vi "Plot SJ Datafile.vi"(11 "File Path Control":path) -> ()   [LabVIEW 2011]
uses:
  <vilib>/Utility/file.llb/Read From Spreadsheet File (string).vi
  <vilib>/Utility/file.llb/Read From Spreadsheet File (DBL).vi
  <vilib>/Analysis/NI_AALBase.lvlib
panel:
  out "Fmax":dbl[](array[numeric])
  in  "Sort?":bool
  out "Selected Data SD":dbl format="%.2e"
  out "All Data SD":dbl format="%.2e"
  out "All Data":cluster{dbl[], dbl[]}[](graph)
  in  "Disc ID List":i32[](listbox)
  out "Selected Data":cluster{dbl[], dbl[]}[](graph)
  # "C:\\EnFlo_Data_Local\\2012\\Aero_Tunnel\\Nick_Martin\\Results_Post_Processed\\SJ_In_RP_Test_I_xls_Mean_Data\\Phase Pressure _deg_.xls"
  # "C:\\EnFlo_Data_Local\\2012\\Aero_Tunnel\\Nick_Martin\\Results_Post_Processed\\SJ_In_RP_Test_I_xls_Mean_Data\\RMS Current _A_.xls"
  # "C:\\EnFlo_Data_Local\\2012\\Aero_Tunnel\\Nick_Martin\\Results_Post_Processed\\SJ_In_RP_Test_I_xls_Mean_Data\\RMS Pressure _Pa_.xls"
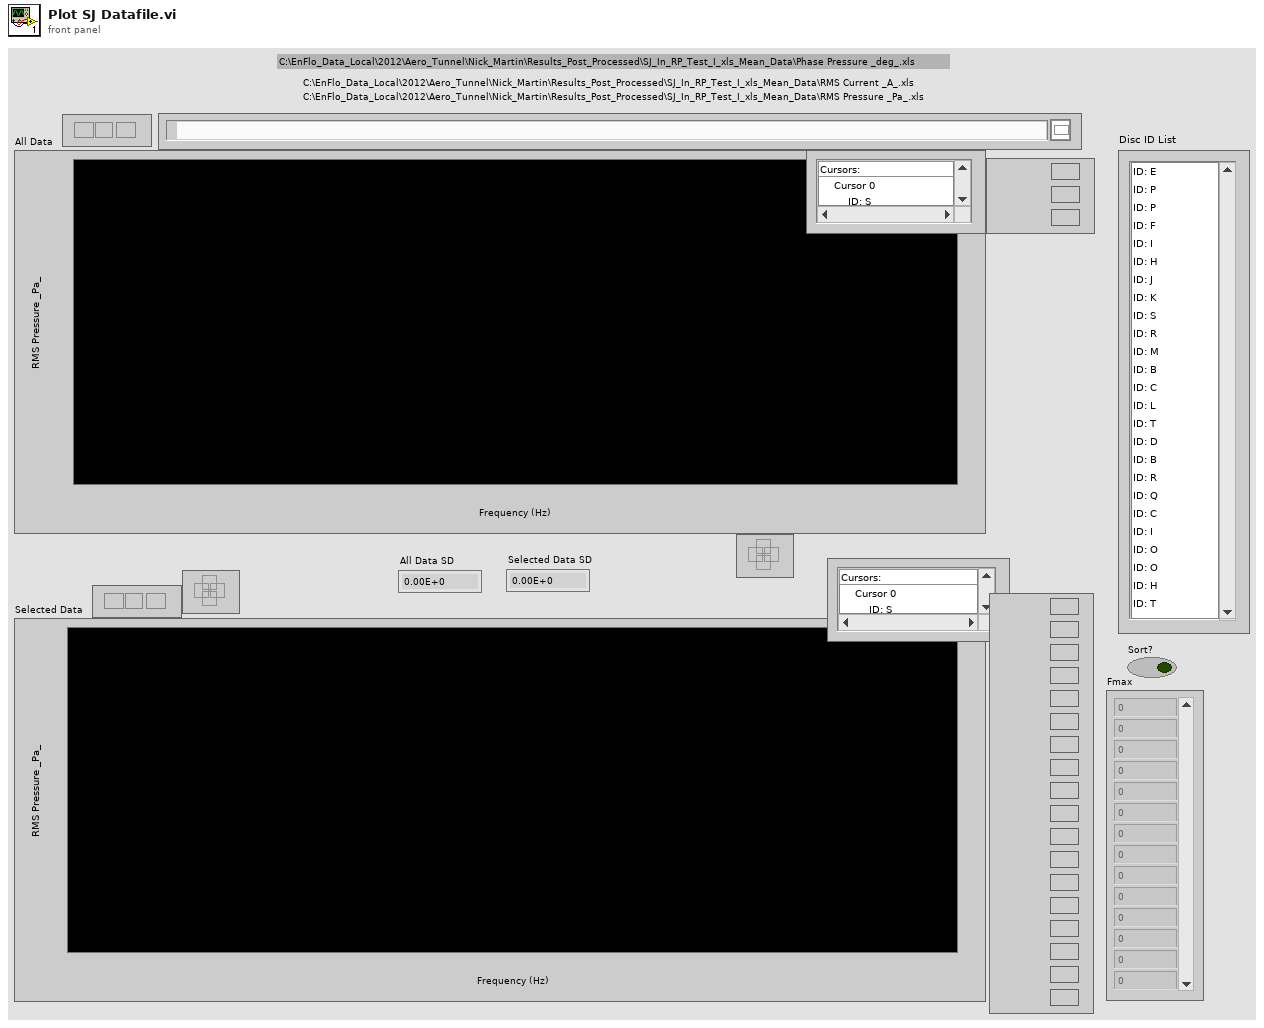
[diagram p1: front panel]
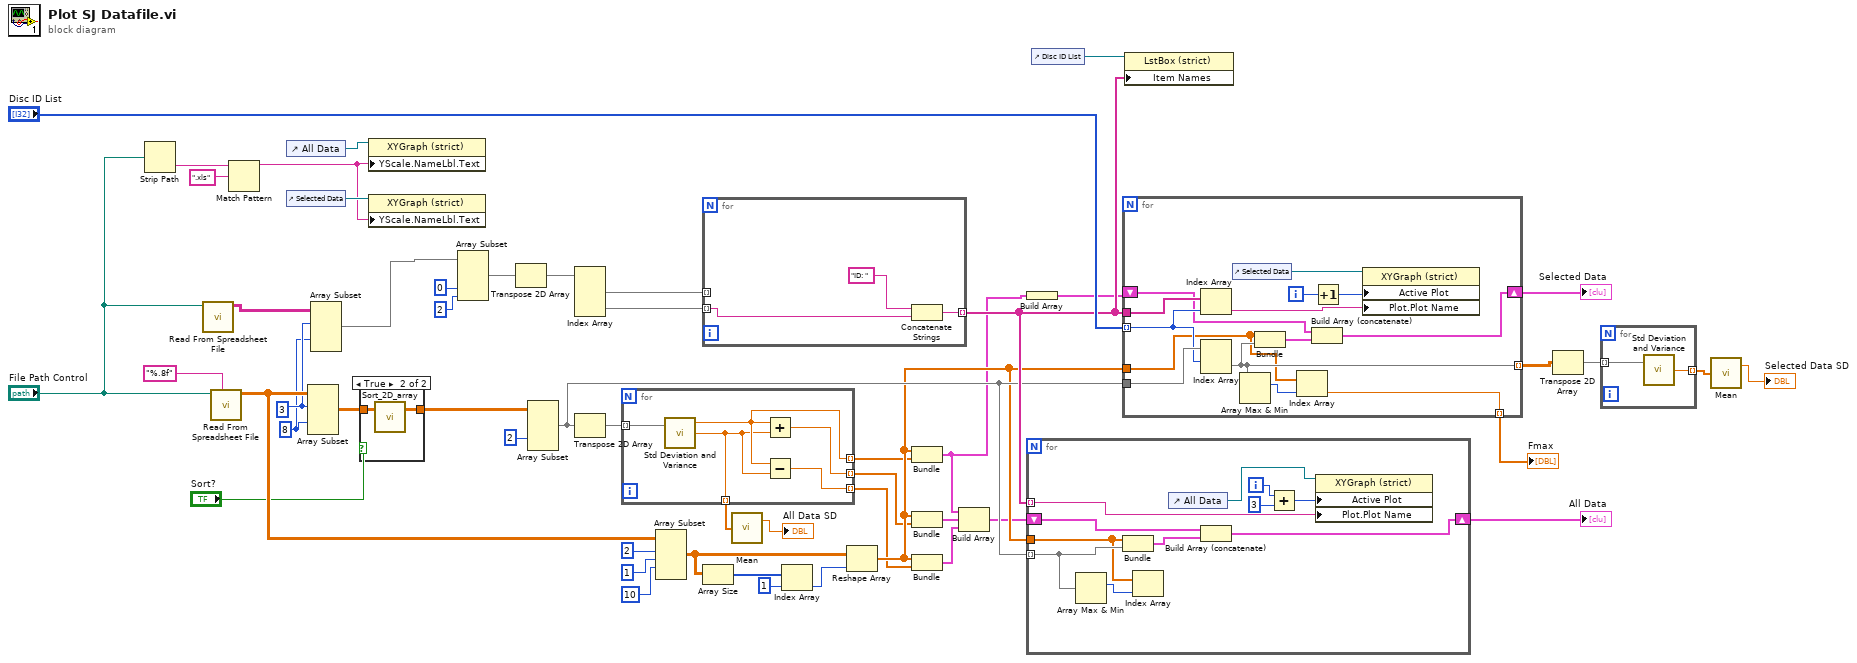
[diagram p0: block diagram]
diagram:
  w8 = 8 ("index")
  w9 = 3 ("index")
  n1 = Strip Path(path="File Path Control") -> (name=w32:string)  [unwired: 1 out]
  n2 = call-poly <vilib>:"Read From Spreadsheet File.vi"("file path (dialog if empty)"="File Path Control") -> ("all rows"=w7:string[][])  [unwired: 6 in, 4 out]
  n3 = call-poly <vilib>:"Read From Spreadsheet File.vi"("format (%.3f)"="%.8f", "file path (dialog if empty)"="File Path Control") -> ("all rows"=w44:dbl[][])  [unwired: 5 in, 4 out]
  n4 = Match Pattern(string=w32, regular expression=".xls") -> (before substring=w28:string)  [unwired: 1 in, 3 out]
  n5 = control-ref of="All Data"() -> (w30:refnum<vi>)
  n6 = control-ref of="Selected Data"() -> (w29:refnum<vi>)
  n7 = Array Subset(array=w44, index (row)=w9, index (col)=w8) -> (w42:dbl[][])  [unwired: 2 in]
  n8 = Array Subset(array=w7, index (row)=w9, index (col)=w8) -> (w5:string[][])  [unwired: 2 in]
  n9 = case shown="True" "Sort?" {
    tunnel: w42 -> [w53 w55]
    tunnel: [w53 w54] -> w4
    frame False {
    }
    frame True {
      n10 = call "Sort_2D_array.vi"("unsorted array"=w55) -> ("sorted array"=w54:dbl[][])  [unwired: 1 in, 1 out]
    }
  }
  n11 = property class="XYGraph (strict)"(reference=w30, "YScale.NameLbl.Text"=w28) -> ()  [unwired: 1 in, 2 out]
  n12 = property class="XYGraph (strict)"(reference=w29, "YScale.NameLbl.Text"=w28) -> ()  [unwired: 1 in, 2 out]
  n13 = Array Subset(array=w5, index (col)=0 ("index"), length (col)=2 ("length")) -> (w39:string[][])  [unwired: 2 in]
  n14 = Transpose 2D Array(2D array=w39) -> (transposed array=w43:string[][])
  n15 = Array Subset(array=w4, index (col)=2 ("index")) -> (w27:dbl[][])  [unwired: 3 in]
  n16 = Index Array(array=w43) -> (element #1=w3:string[], element #2=w2:string[])  [unwired: 4 in]
  n17 = Transpose 2D Array(2D array=w27) -> (transposed array=w26:dbl[][])
  n18 = for {
    tunnel: w26 -> [w60] mode=indexing
    tunnel: [w58] -> w24 mode=indexing
    tunnel: [w59] -> w23 mode=indexing
    tunnel: [w57] -> w22 mode=indexing
    tunnel: [w56] -> w18 mode=indexing
    n19 = call <vilib>:"Std Deviation and Variance.vi"("X"=w60) -> ("mean"=w58:dbl, "standard deviation"=w56:dbl)  [unwired: 1 in, 1 out]
    n20 = Add(x=w58, y=w56) -> (x+y=w59:dbl)
    n21 = Subtract(x=w58, y=w56) -> (x-y=w57:dbl)
  }
  n22 = Array Subset(array=w44, index (row)=2 ("index"), length (row)=1 ("length"), index (col)=10 ("index")) -> (w48:dbl[][])  [unwired: 1 in]
  n23 = for {
    tunnel: w2 -> [w61] mode=indexing
    tunnel: [w62] -> w34 mode=indexing
    tunnel: w3 -> [_] mode=indexing
    n24 = Concatenate Strings("ID: " ("string"), w61) -> (w62:string)
  }
  n25 = Array Size(array=w48) -> (size(s)=w47:i32[])
  n26 = call <vilib>:"Mean.vi"("X"=w18) -> ("mean"=→"All Data SD":dbl)  [unwired: 1 out]
  n27 = Index Array(array=w47, index=1) -> (element=w45:i32)
  n28 = Reshape Array(w48, w45) -> (w25:dbl[])
  n29 = Bundle(w25, w24) -> (w12:cluster{dbl[], dbl[]})  [unwired: 1 in]
  n30 = Bundle(w25, w23) -> (w21:cluster{dbl[], dbl[]})  [unwired: 1 in]
  n31 = Bundle(w25, w22) -> (w20:cluster{dbl[], dbl[]})  [unwired: 1 in]
  n32 = Build Array(w12, w21, w20) -> (w19:cluster{dbl[], dbl[]}[])
  n33 = Build Array(w12) -> (w11:cluster{dbl[], dbl[]}[])
  n34 = for {
    tunnel: w25 -> [w65]
    tunnel: w27 -> [w66] mode=indexing
    shift-right: [w72] -> w33
    shift-left: w19 -> [w71]
    tunnel: w34 -> [w70] mode=indexing
    i -> [w73]
    n35 = Array Max & Min(array=w66) -> (max index (indices)=w64:i32)  [unwired: 3 out]
    n36 = Bundle(w65, w66) -> (w74:cluster{dbl[], dbl[]})  [unwired: 1 in]
    n37 = Index Array(array=w65, index=w64) -> ()  [unwired: 1 out]
    n38 = control-ref of="All Data"() -> (w69:refnum<vi>)
    n39 = Build Array (concatenate)(w71, w74) -> (w72:cluster{dbl[], dbl[]}[])
    n40 = Add(x=w73, y=3) -> (x+y=w68:i32)
    n41 = property class="XYGraph (strict)"(reference=w69, "Active Plot"=w68, "Plot.Plot Name"=w70) -> ()  [unwired: 1 in, 2 out]
  }
  "All Data" <- w33
  n42 = control-ref of="Disc ID List"() -> (w37:refnum<vi>)
  n43 = for {
    tunnel: "Disc ID List" -> [w84] mode=indexing
    tunnel: w25 -> [w76]
    tunnel: w27 -> [w88]
    tunnel: w34 -> [w85]
    shift-right: [w82] -> w35
    shift-left: w11 -> [w81]
    tunnel: [w77] -> w15 mode=indexing
    tunnel: [w75] -> w1 mode=indexing
    i -> [w80]
    n44 = Index Array(array=w85, index=w84) -> (element=w83:string)
    n45 = Index Array(array=w88, index (row)=w84) -> (element=w77:dbl[])  [unwired: 1 in]
    n46 = control-ref of="Selected Data"() -> (w86:refnum<vi>)
    n47 = Array Max & Min(array=w77) -> (max index (indices)=w78:i32)  [unwired: 3 out]
    n48 = Bundle(w76, w77) -> (w87:cluster{dbl[], dbl[]})  [unwired: 1 in]
    n49 = Index Array(array=w76, index=w78) -> (element=w75:dbl)
    n50 = Build Array (concatenate)(w81, w87) -> (w82:cluster{dbl[], dbl[]}[])
    n51 = Increment(x=w80) -> (x+1=w79:i32)
    n52 = property class="XYGraph (strict)"(reference=w86, "Active Plot"=w79, "Plot.Plot Name"=w83) -> ()  [unwired: 1 in, 2 out]
  }
  "Selected Data" <- w35
  "Fmax" <- w1
  n53 = property class="LstBox (strict)"(reference=w37, "Item Names"=w34) -> ()  [unwired: 1 in, 2 out]
  n54 = Transpose 2D Array(2D array=w15) -> (transposed array=w14:dbl[][])
  n55 = for {
    tunnel: w14 -> [w90] mode=indexing
    tunnel: [w89] -> w16 mode=indexing
    n56 = call <vilib>:"Std Deviation and Variance.vi"("X"=w90) -> ("standard deviation"=w89:dbl)  [unwired: 1 in, 2 out]
  }
  n57 = call <vilib>:"Mean.vi"("X"=w16) -> ("mean"=→"Selected Data SD":dbl)  [unwired: 1 out]
